vi "MAAP7.vi"   [LabVIEW 2016]
uses:
  <vilib>/NXT/Block Support/NXT_InputPort.ctl
  <vilib>/NXT/LegoClasses/BrickReference/BrickReference.lvclass
  <vilib>/NXT/Subs/LVHSConnector.ctl
  <vilib>/NXT/Block Support/NXT_OutputPort.ctl
  <vilib>/NXT/NXTIO Xnodes/NXTIONodeSubVIs/NXTMoveMotors.vi
  <vilib>/NXT/NXTIO Xnodes/NXTIOXNode/NXTIO.xnode
  <vilib>/NXT/NXTIO Xnodes/NXTIONodeSubVIs/LEGOStopAllMotors.vi
  <vilib>/NXT/NXTIO Xnodes/AddressXNode/NXTIOAddress.xnode
  <vilib>/NXT/Dual Mode Library/Sound/PlayC.vi
  <vilib>/NXT/Dual Mode Library/Sensors/Light_On.vi
types:
  T1 = typedef "LVHSConnector.ctl" = refnum<class "BrickReference.lvclass">
  T2 = typedef "NXT_InputPort.ctl" = u32
  T3 = typedef "NXT_OutputPort.ctl" = u8
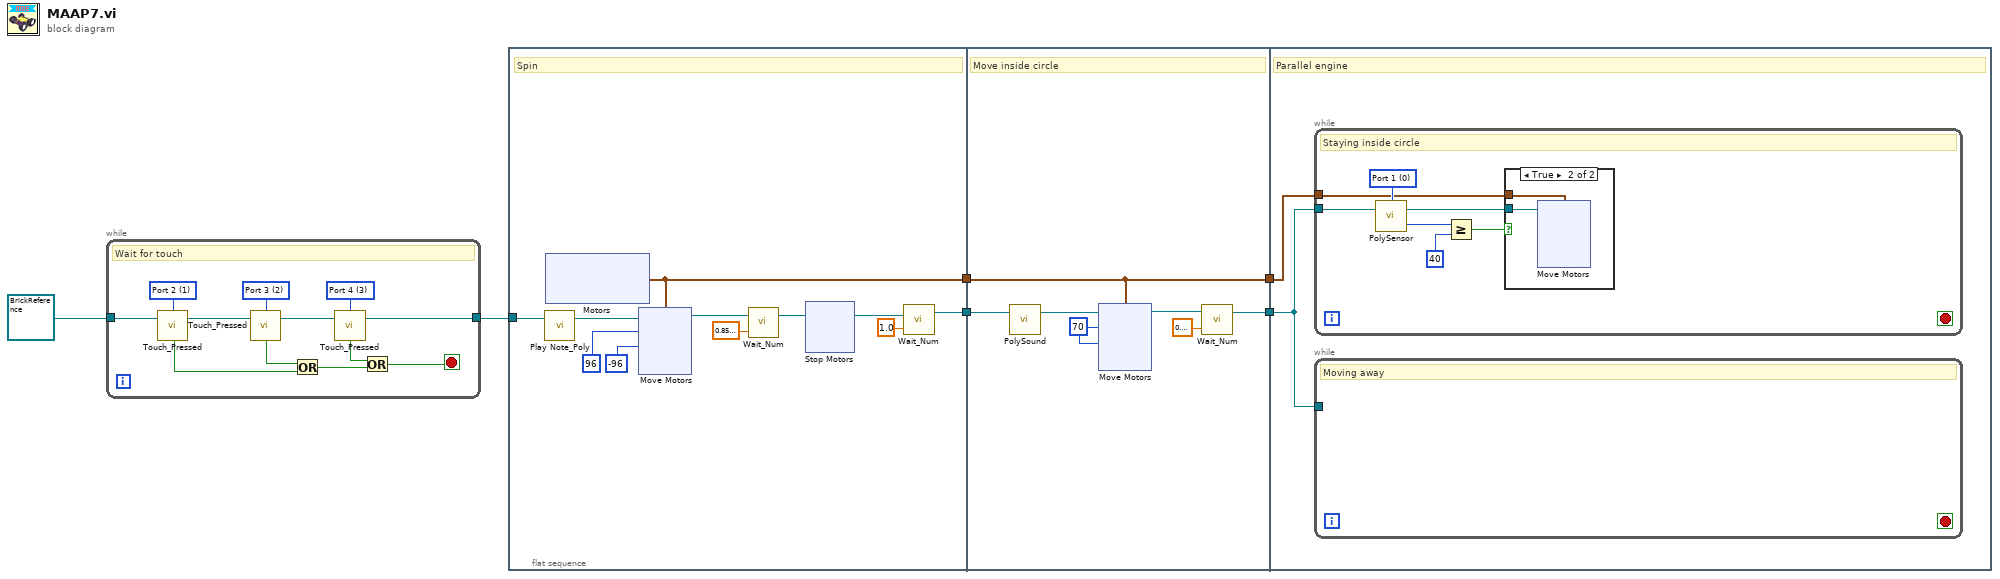
[diagram p0: block diagram]
diagram:
  n1 = while {
    tunnel: [w8] -> w5
    tunnel: T1 refnum ("NXT/EV3") -> [w7]
    stop <- w9 stop-if-true
    w14 = T2 3 items=["Port 1", "Port 2", "Port 3", "Port 4"] ("Port (Port 1)")
    w16 = T2 2 items=["Port 1", "Port 2", "Port 3", "Port 4"] ("Port (Port 1)")
    w18 = T2 1 items=["Port 1", "Port 2", "Port 3", "Port 4"] ("Port (Port 1)")
    # "Wait for touch"
    n2 = call <vilib>:"Touch_Pressed.vi"("NXT/EV3"=w7, "Port (Port 1)"=w18) -> ("Yes / No"=w12:bool, "NXT/EV3"=w17:T1)  [unwired: 1 in]
    n3 = call <vilib>:"Touch_Pressed.vi"("NXT/EV3"=w17, "Port (Port 1)"=w16) -> ("Yes / No"=w13:bool, "NXT/EV3"=w15:T1)  [unwired: 1 in]
    n4 = Or(x=w13, y=w12) -> (x .or. y?=w11:bool)
    n5 = call <vilib>:"Touch_Pressed.vi"("NXT/EV3"=w15, "Port (Port 1)"=w14) -> ("Yes / No"=w10:bool, "NXT/EV3"=w8:T1)  [unwired: 1 in]
    n6 = Or(x=w10, y=w11) -> (x .or. y?=w9:bool)
  }
  n7 = flat-sequence {
    tunnel: w5 -> [w26]
    tunnel: [w20] -> w4
    tunnel: [w19] -> w3
    tunnel: w4 -> [w46]
    tunnel: w3 -> [w42]
    tunnel: [w43] -> w2
    tunnel: [w42] -> w1
    tunnel: w2 -> [w58]
    tunnel: w1 -> [w57]
    frame #0 {
      # "Spin"
      n8 = call-poly <vilib>:"Play Note_Poly.vi"("NXT/EV3"=w26) -> ("NXT/EV3"=w25:T1)  [unwired: 3 in]
      n9 = xnode "Motors"() -> ("Motor"=w19:cluster{"Port":T3, "Port":T3})
      n10 = xnode "Move Motors"("Power/Speed 2"=i8 -96, "Power/Speed 1"=i8 96, "Motors"=w19, "NXT/EV3"=w25) -> ("NXT/EV3"=w24:T1)
      n11 = call <vilib>:"Wait_Num.vi"("Time (1 sec)"=sgl 0.85, "NXT/EV3"=w24) -> ("NXT/EV3"=w27:T1)  [unwired: 2 in]
      n12 = xnode "Stop Motors"("NXT/EV3"=w27) -> ("NXT/EV3"=w23:T1)  [unwired: 1 in]
      n13 = call <vilib>:"Wait_Num.vi"("Time (1 sec)"=sgl 1.0, "NXT/EV3"=w23) -> ("NXT/EV3"=w20:T1)  [unwired: 2 in]
    }
    frame #1 {
      w45 = i8 70 ("Power/Speed 1")
      # "Move inside circle"
      n14 = call-poly <vilib>:"PolySound.vi"("NXT/EV3"=w46) -> ("NXT/EV3"=w44:T1)  [unwired: 3 in]
      n15 = xnode "Move Motors"("Power/Speed 2"=w45, "Power/Speed 1"=w45, "Motors"=w42, "NXT/EV3"=w44) -> ("NXT/EV3"=w47:T1)
      n16 = call <vilib>:"Wait_Num.vi"("Time (1 sec)"=sgl 0.7, "NXT/EV3"=w47) -> ("NXT/EV3"=w43:T1)  [unwired: 2 in]
    }
    frame #2 {
      # "Parallel engine"
      n17 = while {
        tunnel: w58 -> [w65]
        tunnel: w57 -> [w60]
        stop <- _ stop-if-true
        w64 = T2 0 items=["Port 1", "Port 2", "Port 3", "Port 4"] ("Port (Port 1)")
        # "Staying inside circle"
        n18 = call-poly <vilib>:"PolySensor.vi"("NXT/EV3"=w65, "Port (Port 3)"=w64) -> ("Scaled Value"=w63:i16, "NXT/EV3"=w61:T1)  [unwired: 1 in]
        n19 = Greater Or Equal?(x=w63, y=i16 40) -> (x >= y?=w59:bool)
        n20 = case shown="True" w59 {
          tunnel: w61 -> [_ w67]
          tunnel: w60 -> [_ w66]
          frame False {
          }
          frame True {
            n21 = xnode "Move Motors"("Motors"=w66, "NXT/EV3"=w67) -> ()  [unwired: 2 in, 1 out]
          }
        }
      }
      n22 = while {
        tunnel: w58 -> [_]
        stop <- _ stop-if-true
        # "Moving away"
      }
    }
  }
